vi "Create Same Type Image v2.vi"(8 "error in (no error)":errorcluster, 9 "Name in":string, 10 "Image Dst":T1, 11 "Image Src":T1) -> (0 "error out":errorcluster, 1 "Name out":string, 2 "Image Dst":T1)   [LabVIEW 2021]
uses:
  <vilib>/vision/Image Controls.llb/IMAQ Image.ctl
panel:
  out "Message":string
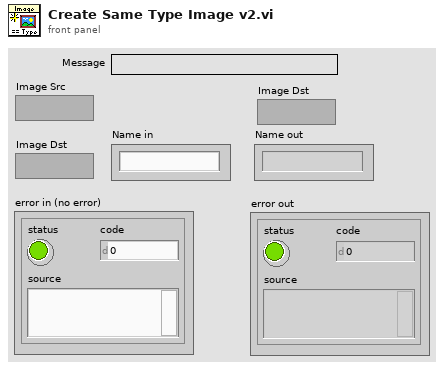
[diagram p1: front panel]
types:
  T1 = typedef "IMAQ Image.ctl" = refnum<image>
  T2 = typedef "Image Type" = u32
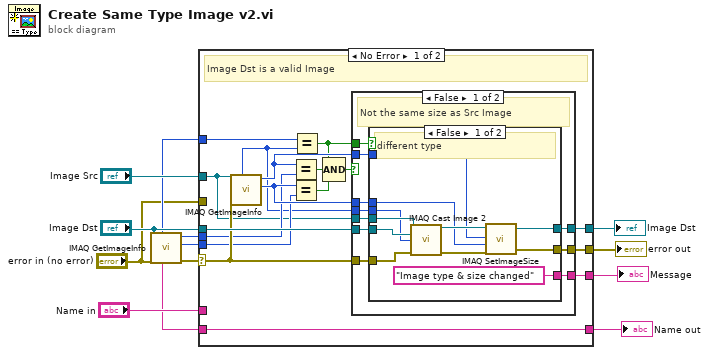
[diagram p0: block diagram]
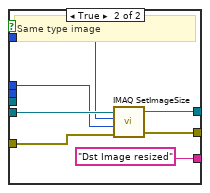
[diagram p2: hidden frame]
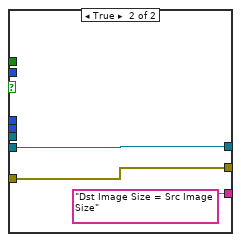
[diagram p3: hidden frame]
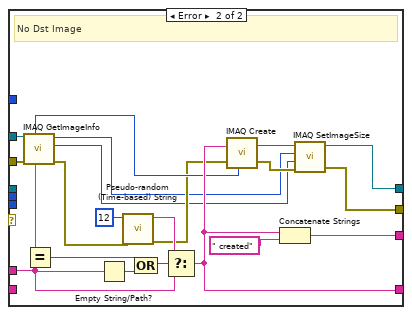
[diagram p4: hidden frame]
diagram:
  n1 = call "IMAQ GetImageInfo"("error in (no error)"="error in (no error)", "Image"="Image Dst") -> ("error out"=w6:errorcluster, "Y Resolution"=w5:i32, "X Resolution"=w4:i32, "Image Name"=w2:string, "Image Type"=w3:T2)  [unwired: 2 in, 3 out]
  n2 = case shown="No Error" w6 {
    selector: w6 -> [w21 _]
    tunnel: "Image Src" -> [w16 w81]
    tunnel: "Name in" -> [_ w73]
    tunnel: [w25 w74] -> w11
    tunnel: [w14 w80] -> w10
    tunnel: [w26 w76] -> w9
    tunnel: "Image Dst" -> [w27 _]
    tunnel: [w22 w78] -> w8
    tunnel: w5 -> [w20 _]
    tunnel: w4 -> [w19 _]
    tunnel: w3 -> [w18 _]
    tunnel: w2 -> [w14 _]
    tunnel: "error in (no error)" -> [_ w68]
    frame No Error {
      # "Image Dst is a valid Image"
      n3 = call "IMAQ GetImageInfo"("error in (no error)"=w21, "Image"=w16) -> ("Y Resolution"=w23:i32, "X Resolution"=w24:i32, "Image Type"=w15:T2)  [unwired: 2 in, 5 out]
      n4 = Equal?(x=w24, y=w19) -> (x = y?=w30:bool)
      n5 = Equal?(x=w23, y=w20) -> (x = y?=w29:bool)
      n6 = Equal?(x=w18, y=w15) -> (x = y?=w17:bool)
      n7 = Compound Arithmetic op=AND(w17, w30, w29) -> (w28:bool)
      n8 = case shown="False" w28 {
        tunnel: w27 -> [w40 w61]
        tunnel: [w39 w61] -> w26
        tunnel: [w38 w59] -> w25
        tunnel: w24 -> [w37 _]
        tunnel: w23 -> [w36 _]
        tunnel: w21 -> [w35 w59]
        tunnel: [w34 "Dst Image Size = Src Image Size"] -> w22
        tunnel: w17 -> [w33 _]
        tunnel: w16 -> [w32 _]
        tunnel: w15 -> [w31 _]
        frame False {
          # "Not the same size as Src Image"
          n9 = case shown="False" w33 {
            tunnel: w40 -> [w50 w58]
            tunnel: [w43 w57] -> w39
            tunnel: [w46 w56] -> w38
            tunnel: w37 -> [w45 w55]
            tunnel: w36 -> [w44 w54]
            tunnel: w35 -> [w49 w53]
            tunnel: ["Image type & size changed" "Dst Image resized"] -> w34
            tunnel: w32 -> [w51 _]
            tunnel: w31 -> [w41 _]
            frame False {
              # "different type"
              n10 = call "IMAQ Cast Image 2"("Image Src"=w51, "Image Dst"=w50, "Image Type"=w41, "error in (no error)"=w49) -> ("Image Dst Out"=w48:T1, "error out"=w47:errorcluster)  [unwired: 10 in]
              n11 = call "IMAQ SetImageSize"("error in (no error)"=w47, "Y Resolution"=w44, "X Resolution"=w45, "Image"=w48) -> ("error out"=w46:errorcluster, "Image Out"=w43:T1)  [unwired: 1 in]
            }
            frame True {
              # "Same type image"
              n12 = call "IMAQ SetImageSize"("error in (no error)"=w53, "Y Resolution"=w54, "X Resolution"=w55, "Image"=w58) -> ("error out"=w56:errorcluster, "Image Out"=w57:T1)  [unwired: 1 in]
            }
          }
        }
        frame True {
        }
      }
    }
    frame Error {
      # "No Dst Image"
      n13 = call "IMAQ GetImageInfo"("error in (no error)"=w68, "Image"=w81) -> ("error out"=w66:errorcluster, "Y Resolution"=w62:i32, "X Resolution"=w63:i32, "Image Name"=w72:string, "Image Type"=w69:T2)  [unwired: 2 in, 3 out]
      n14 = Equal?(x=w72, y=w73) -> (x = y?=w71:bool)
      n15 = Empty String/Path?(string/path=w73) -> (empty?=w70:bool)
      n16 = call "Pseudo-random (Time-based) String.vi"("Error In"=w66, "Length (10)"=u32 12) -> ("Error Out"=w65:errorcluster, "result string"=w67:string)  [unwired: 8 in]
      n17 = Compound Arithmetic op=OR(w71, w70) -> (w77:bool)
      n18 = Select(t=w67, s=w77, f=w73) -> (s? t:f=w80:string)
      n19 = call "IMAQ Create"("Image Name"=w80, "Image Type"=w69, "error in (no error)"=w65) -> ("New Image"=w76:T1, "error out"=w75:errorcluster)  [unwired: 2 in]
      n20 = Concatenate Strings(w80, " created" ("string")) -> (w78:string)
      n21 = call "IMAQ SetImageSize"("error in (no error)"=w75, "Y Resolution"=w62, "X Resolution"=w63, "Image"=w76) -> ("error out"=w74:errorcluster)  [unwired: 1 in, 1 out]
    }
  }
  "error out" <- w11
  "Image Dst" <- w9
  "Name out" <- w10
  "Message" <- w8
